vi "CopyAllData.vi"(8 "error in (no error)":errorcluster) -> (0 "error out":errorcluster, 1 "pData2":u16[](array[numeric]), 2 "pData1":u16[](array[numeric]))   [LabVIEW 2015, in "ESLSCDLL.lvlib"]
uses:
  ESLSCDLL.lvlib
  Globals.vi
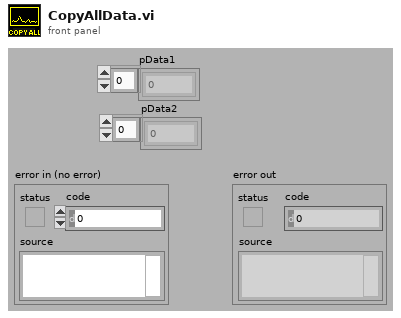
[diagram p1: front panel]
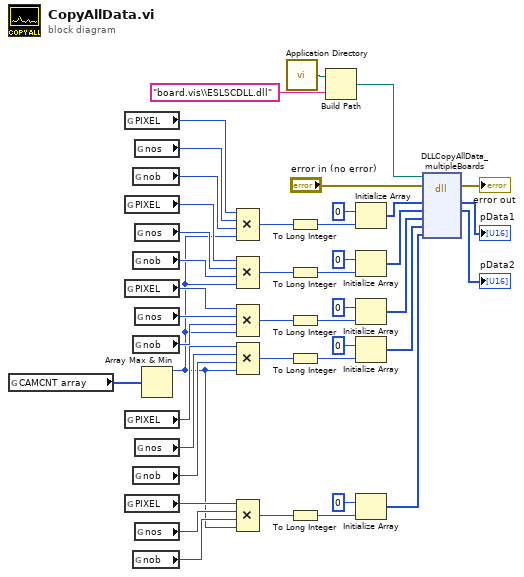
[diagram p0: block diagram]
diagram:
  n1 = global read "Globals.vi" "CAMCNT array"() -> (w23:u32[])
  n2 = global read "Globals.vi" "PIXEL"() -> (w37:u32)
  n3 = global read "Globals.vi" "PIXEL"() -> (w30:u32)
  n4 = global read "Globals.vi" "PIXEL"() -> (w19:u32)
  n5 = global read "Globals.vi" "PIXEL"() -> (w13:u32)
  n6 = global read "Globals.vi" "PIXEL"() -> (w7:u32)
  n7 = global read "Globals.vi" "nob"() -> (w36:u32)
  n8 = global read "Globals.vi" "nob"() -> (w29:u32)
  n9 = global read "Globals.vi" "nob"() -> (w18:u32)
  n10 = global read "Globals.vi" "nob"() -> (w12:u32)
  n11 = global read "Globals.vi" "nob"() -> (w6:u32)
  n12 = global read "Globals.vi" "nos"() -> (w35:u32)
  n13 = global read "Globals.vi" "nos"() -> (w28:u32)
  n14 = global read "Globals.vi" "nos"() -> (w17:u32)
  n15 = global read "Globals.vi" "nos"() -> (w11:u32)
  n16 = global read "Globals.vi" "nos"() -> (w5:u32)
  n17 = Array Max & Min(array=w23) -> (max value=w4:u32)  [unwired: 3 out]
  n18 = Compound Arithmetic op=MULTIPLY(w37, w35, w36, w4) -> (w38:u32)
  n19 = Compound Arithmetic op=MULTIPLY(w30, w28, w29, w4) -> (w31:u32)
  n20 = Compound Arithmetic op=MULTIPLY(w19, w17, w18, w4) -> (w20:u32)
  n21 = Compound Arithmetic op=MULTIPLY(w13, w11, w12, w4) -> (w14:u32)
  n22 = Compound Arithmetic op=MULTIPLY(w7, w5, w6, w4) -> (w8:u32)
  n23 = call <vilib>:"Application Directory.vi"() -> ("Application Directory"=w43:path)
  n24 = To Long Integer(number=w38) -> (32bit integer=w40:i32)
  n25 = To Long Integer(number=w31) -> (32bit integer=w33:i32)
  n26 = To Long Integer(number=w20) -> (32bit integer=w22:i32)
  n27 = To Long Integer(number=w14) -> (32bit integer=w16:i32)
  n28 = To Long Integer(number=w8) -> (32bit integer=w10:i32)
  n29 = Build Path(base path=w43, name or relative path="board.vis\\ESLSCDLL.dll") -> (appended path=w41:path)
  n30 = Initialize Array(u16 0, w40) -> (w34:u16[])
  n31 = Initialize Array(u16 0, w33) -> (w27:u16[])
  n32 = Initialize Array(u16 0, w22) -> (w3:u16[])
  n33 = Initialize Array(u16 0, w16) -> (w2:u16[])
  n34 = Initialize Array(u16 0, w10) -> (w1:u16[])
  n35 = dll-call lib="C:/ENTW/PCIE/LV64/board.vis/ESLSCDLL.dll" fn="DLLCopyAllData_multipleBoards" ("lwlscdll.dll:DLLReadLongS0")(path in=w41, error in="error in (no error)", "pdest0"=w34, "pdest1"=w27, "pdest2"=w3, "pdest3"=w2, "pdest4"=w1) -> (error out=→"error out":errorcluster, "pdest0"=→"pData1":u16[], "pdest1"=→"pData2":u16[])  [unwired: 5 in, 1 out]
